vi "Extract Newest with minimum duration.vi"(4 "Force Duration":bool, 6 "Duration(S)":dbl, 8 "Error":errorcluster, 9 "Pointer":refnum<class "_Pointer.lvclass">, 10 "Index":i32=-1, 11 "WavBuf":refnum<class "WavBuf.lvclass">) -> (0 "Error Out":errorcluster, 2 "Waveform Out":T1, 3 "WavBuf Out":refnum<class "WavBuf.lvclass">)   [LabVIEW 2024, in "WavBuf.lvclass"]
uses:
  WavBuf.lvclass
  Universal Controls/Waveform_Data.ctl
  Pointer/_Pointer.lvclass
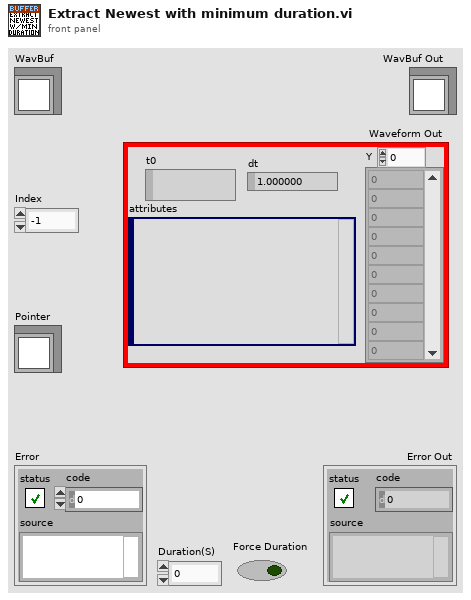
[diagram p1: front panel]
types:
  T1 = typedef "Waveform_Data.ctl" = waveform(dbl)
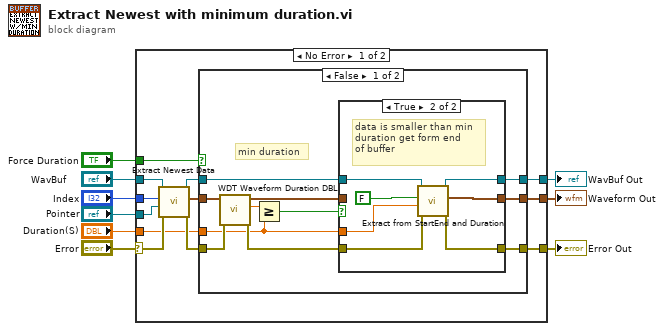
[diagram p0: block diagram]
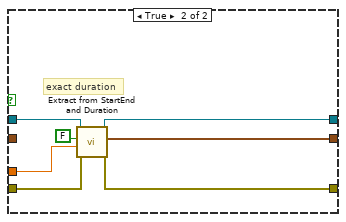
[diagram p3: hidden frame]
diagram:
  n1 = case shown="No Error" "Error" {
    selector: "Error" -> [w18 w51]
    tunnel: [w14 w51] -> w8
    tunnel: [w12 w50] -> w6
    tunnel: "WavBuf" -> [w21 w50]
    tunnel: [w15 _] -> w5
    tunnel: "Pointer" -> [w19 _]
    tunnel: "Index" -> [w20 _]
    tunnel: "Duration(S)" -> [w13 _]
    tunnel: "Force Duration" -> [w10 _]
    frame No Error {
      n2 = call "Extract Newest Data.vi"("Error"=w18, "Name"=w19, "Index"=w20, "WavBuf"=w21) -> ("Error Out"=w16:errorcluster, "Newest Data Out"=w17:T1, "WavBuf Out"=w11:refnum<class "WavBuf.lvclass">)  [unwired: 5 in]
      n3 = case shown="False" w10 {
        tunnel: w17 -> [w32 _]
        tunnel: w16 -> [w30 w44]
        tunnel: [w29 w45] -> w15
        tunnel: [w27 w43] -> w14
        tunnel: w13 -> [w25 w49]
        tunnel: [w24 w46] -> w12
        tunnel: w11 -> [w23 w47]
        frame False {
          # "min duration"
          n4 = call <vilib>:"WDT Waveform Duration DBL.vi"("error in (no error)"=w30, "waveform in"=w32) -> ("error out"=w26:errorcluster, "duration"=w31:dbl, "waveform out"=w28:waveform(dbl))  [unwired: 7 out]
          n5 = Greater Or Equal?(x=w31, y=w25) -> (x >= y?=w22:bool)
          n6 = case shown="True" w22 {
            tunnel: [w35 w38] -> w29
            tunnel: w28 -> [w35 _]
            tunnel: [w34 w39] -> w27
            tunnel: w26 -> [w34 w40]
            tunnel: w25 -> [_ w37]
            tunnel: [w33 w41] -> w24
            tunnel: w23 -> [w33 w42]
            frame False {
              # "data is larger than\nmin duration send all"
            }
            frame True {
              # "data is smaller than min \nduration get form end \nof buffer"
              n7 = call "Extract from StartEnd and Duration.vi"("Error"=w40, "Duration(S)"=w37, "From End(f)\nFrom Beginning(t)"=FALSE ("From End(f)\nFrom Beginning(t)"), "WavBuf"=w42) -> ("Error Out"=w39:errorcluster, "Waveform Out"=w38:T1, "WavBuf Out"=w41:refnum<class "WavBuf.lvclass">)  [unwired: 5 in]
            }
          }
        }
        frame True {
          # "exact duration"
          n8 = call "Extract from StartEnd and Duration.vi"("Error"=w44, "Duration(S)"=w49, "From End(f)\nFrom Beginning(t)"=FALSE ("From End(f)\nFrom Beginning(t)"), "WavBuf"=w47) -> ("Error Out"=w43:errorcluster, "Waveform Out"=w45:T1, "WavBuf Out"=w46:refnum<class "WavBuf.lvclass">)  [unwired: 5 in]
        }
      }
    }
    frame Error {
    }
  }
  "Error Out" <- w8
  "WavBuf Out" <- w6
  "Waveform Out" <- w5
